vi "DAQX mod 1SDI v03.vi"(0 "resource name":refnum<k15>="PXI1Slot2", 1 "close (T)":bool=TRUE, 2 "Record Data":bool, 3 "numSamples":i32=-1, 4 "max time (s)":dbl=10.0 caption="max time", 5 "min sample rate":dbl=100000000.0, 6 "File location":path, 7 "error in":errorcluster, 8 "reference position":dbl=50.0, 9 "Additional text":string, 10 "Type of measurement":T2, 11 "Name root":string, 12 "Record TDMS":bool=TRUE caption="Enable", 13 "channel parameters":T4(array[cluster])=[{"channel name"="0", "input impedance"=0, "maximum input frequency"=30000000.0, "vertical coupling"=1, "probe attenuation"=1.0, "vertical range"=2.0, "vertical offset"=0.0, "channel enabled"=TRUE}, {"channel name"="1", "input impedance"=0, "maximum input frequency"=30000000.0, "vertical coupling"=1, "probe attenuation"=1.0, "vertical range"=2.0, "vertical offset"=0.0, "channel enabled"=TRUE}] {"input impedance" items=["1 mega ohm"=0, "50 ohms"=2]; "vertical coupling" items=["AC", "DC", "Ground"]}, 15 "reset sn":bool) -> (17 "Saving Data":bool, 18 "wfm out":waveform(dbl)[](array[waveform]), 19 "Filename Out":path, 22 "Parameters values file":string, 24 "actualSamples 0":i32, 26 "actualSamples 1":i32, 27 "error out":errorcluster caption="error out final")   [LabVIEW 2013]
doc: "Configures and acquires data from an NI-SCOPE high-speed digitizer.\n--------------------\n\nThis Express VI is configured as follows:\n\nDevice: PXI1Slot2 (PXI-5122)\nSample Rate (S/s): 100M\nRecord length: 2k\nAcquisition Mode: N Samples\nChannel 0\n - Range (V): 2\n - Offset (V): 0\n - Probe attenuation: 1\n - Coupling: \n - Input impedence: 1 \n - Bandwidth (Hz): 0\nChannel 1\n - Range (V): 2\n - Offset (V): 0\n - Probe attenuation: 1\n - Coupling: \n - Input impedence: 1 \n - Bandwidth (Hz): 0\nImmediate"
uses:
  <instrlib>/niScope/Controls/niScope vertical coupling.ctl
  Strict Type Defs/type_meas_enum.ctl
  <instrlib>/niScope/Controls/niScope timestamp type.ctl
  <instrlib>/niScope/Acquire/Fetch/niScope Multi Fetch Binary 16.vi
  <instrlib>/niScope/Acquire/Fetch/niScope Multi Fetch WDT.vi
  <instrlib>/niScope/Configure/Trigger/niScope Configure Trigger Immediate.vi
  Global VIs/shotnoise.vi
panel:
  out "Chan 1 params":T1
  out "Chan 0 params":T1
  out "file location into parameter files":path
  out "size(s)":i32
  out "actual sample rate":dbl
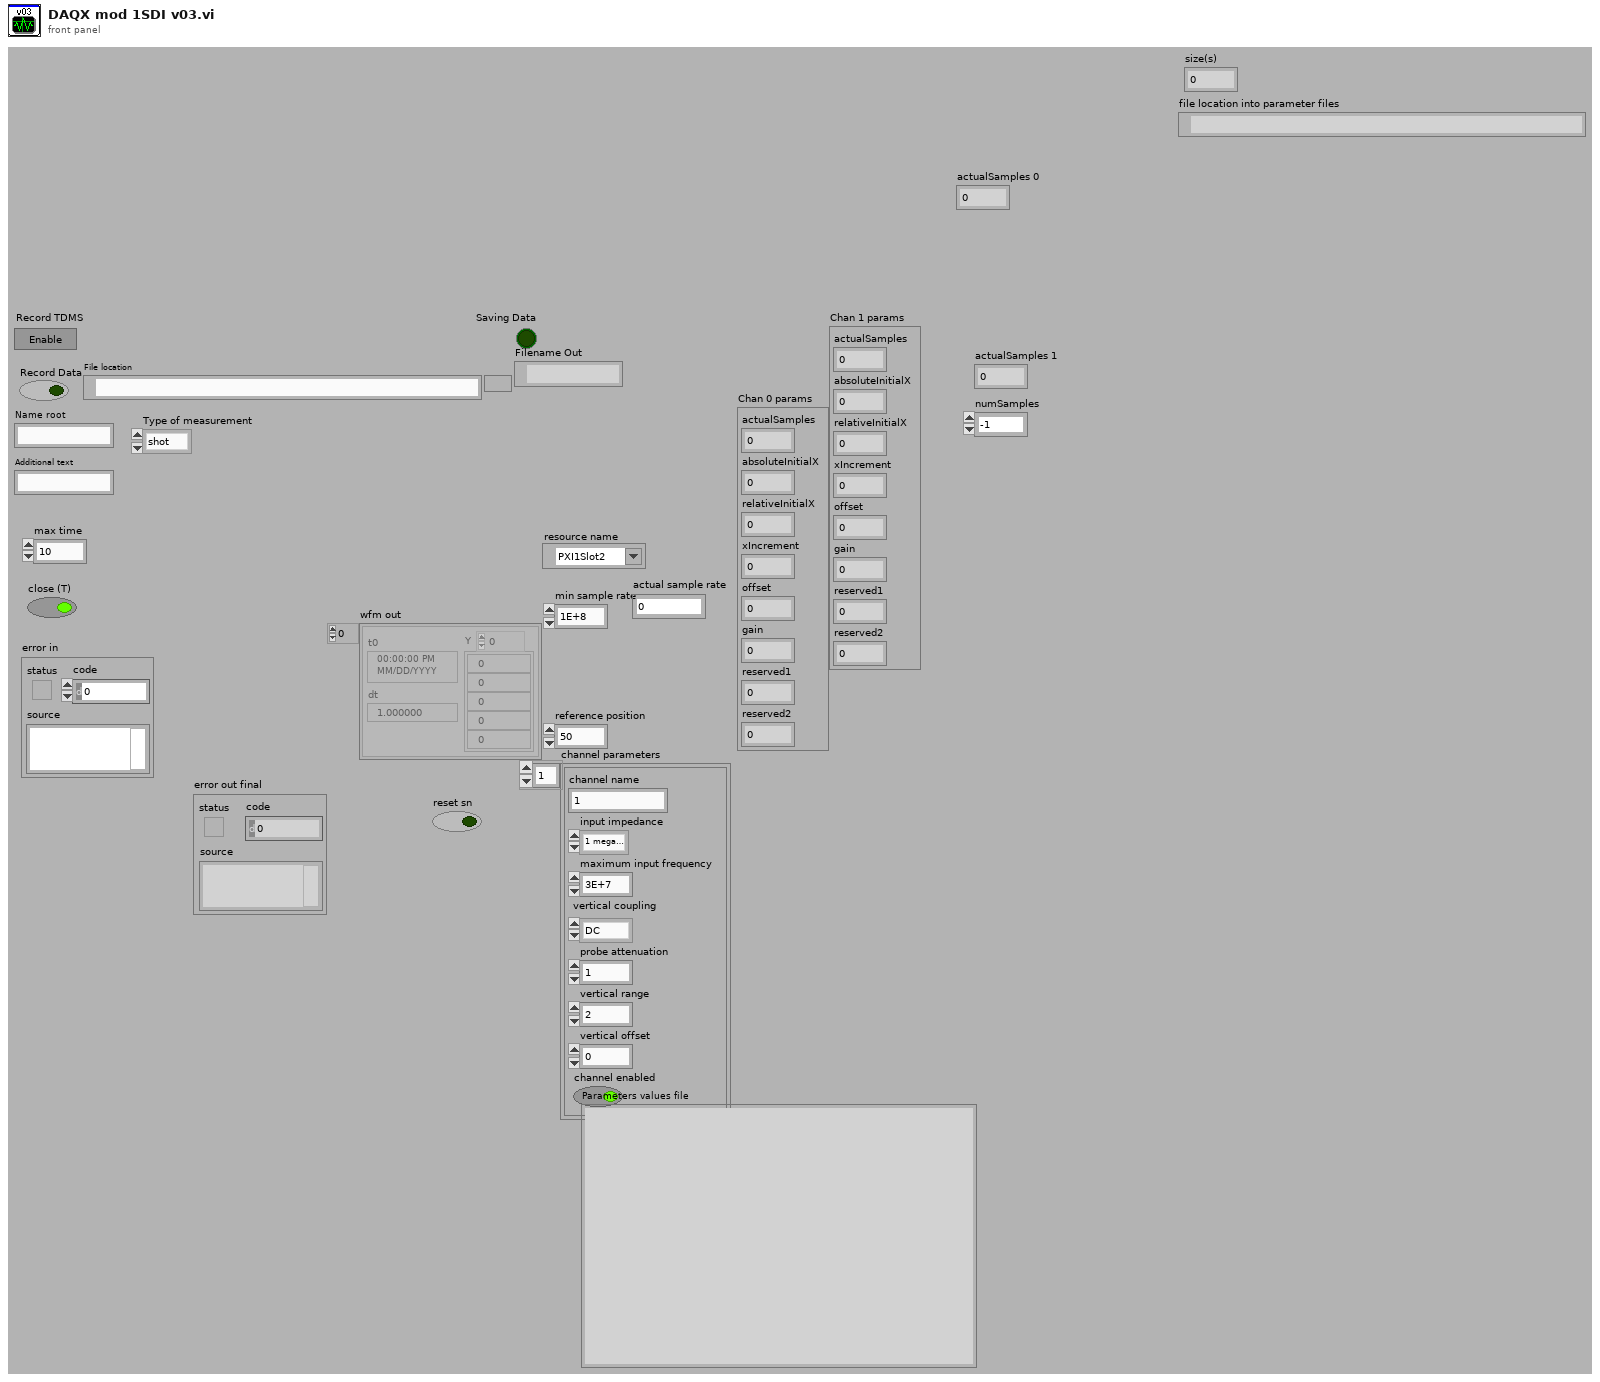
[diagram p1: front panel]
types:
  T1 = cluster{"actualSamples":i32, "absoluteInitialX":dbl, "relativeInitialX":dbl, "xIncrement":dbl, "offset":dbl, "gain":dbl, "reserved1":dbl, "reserved2":dbl}
  T2 = typedef "type_meas_enum.ctl" = enum16{"shot", "x", "p", "electronic"}
  T3 = typedef "niScope vertical coupling.ctl" = i32
  T4 = cluster{"channel name":string, "input impedance":u32, "maximum input frequency":dbl, "vertical coupling":T3, "probe attenuation":dbl, "vertical range":dbl, "vertical offset":dbl, "channel enabled":bool}[]
  T5 = typedef "niScope timestamp type.ctl" = i32
  T6 = cluster{"actualSamples":i32, "absoluteInitialX":dbl, "relativeInitialX":dbl, "xIncrement":dbl, "offset":dbl, "gain":dbl, "reserved1":dbl, "reserved2":dbl}[]
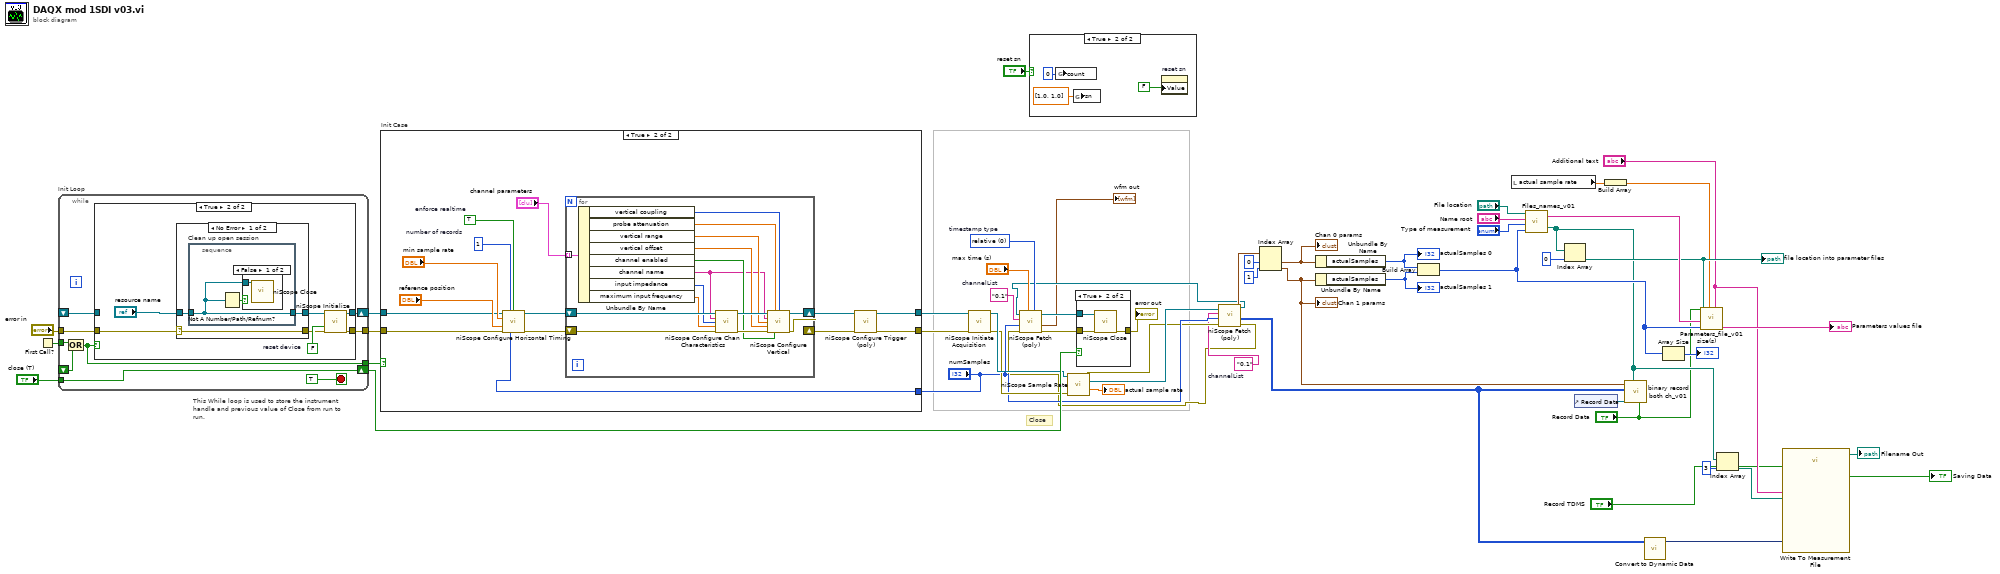
[diagram p0: block diagram]
diagram:
  w18 = "0,1"  # channelList
  w50 = T5 0 items=["relative", "absolute"]  # timestamp type
  w53 = "0,1"  # channelList
  # "This While loop is used to store the instrument handle and previous value of Close from run to run."
  # "Close"
  n1 = First Call?() -> (First Call?: T/F=w49:bool)
  n2 = while "Init Loop" {
    tunnel: w49 -> [w64]
    shift-right: [w63] -> w45
    shift-left: _ -> [w60]
    tunnel: "close (T)" -> [w63]
    shift-right: [w62] -> w48
    shift-left: _ -> [w61]
    tunnel: [w58] -> w47
    tunnel: "error in" -> [w57]
    tunnel: [w56] -> w46
    stop <- TRUE ("stopInit") stop-if-true
    n3 = Or(x=w64, y=w60) -> (x .or. y?=w56:bool)
    n4 = case "Select_Init" shown="True" w56 {
      tunnel: [w66 w71] -> w62
      tunnel: w61 -> [w66 _]
      tunnel: [w65 w70] -> w58
      tunnel: w57 -> [w65 w69]
      frame False {
      }
      frame True {
        w72 = FALSE  # reset device
        n5 = case shown="No Error" w69 {
          selector: w69 -> [w74 w80]
          tunnel: [w76 w81] -> w73
          tunnel: "resource name" -> [w75 w81]
          tunnel: [w74 w80] -> w68
          frame No Error {
            n6 = stacked-sequence "Clean up open session" {
              tunnel: w75 -> [w77]
              tunnel: [w77] -> w76
              frame #0 {
                n7 = Not A Number/Path/Refnum?(number/path/refnum=w77) -> (NaN/Path/Refnum?=w78:bool)
                n8 = case shown="False" w78 {
                  tunnel: w77 -> [w79 _]
                  frame False {
                    n9 = call <instrlib>:"niScope Close.vi"("instrument handle"=w79) -> ()  [unwired: 1 in, 14 out]
                  }
                  frame True {
                  }
                }
              }
            }
          }
          frame Error {
          }
        }
        n10 = call <instrlib>:"niScope Initialize.vi"("resource name"=w73, "reset device"=w72, "error in"=w68) -> ("instrument handle"=w71:refnum<k15>, "error out"=w70:errorcluster)  [unwired: 2 in, 9 out]
      }
    }
  }
  n11 = case "Init Case" shown="True" w46 {
    tunnel: w47 -> [w82 w88]
    tunnel: [w82 w90] -> w52
    tunnel: [w83 w91] -> w51
    tunnel: w48 -> [w83 w89]
    tunnel: "numSamples" -> [_ w84]
    frame False {
    }
    frame True {
      w96 = 1  # number of records
      w97 = TRUE  # enforce realtime
      n12 = call <instrlib>:"niScope Configure Horizontal Timing.vi"("instrument handle"=w89, "number of records"=w96, "enforce realtime"=w97, "min sample rate"="min sample rate", "reference position"="reference position", "error in"=w88, "min record length"=w84) -> ("instrument handle out"=w92:refnum<k15>, "error out"=w93:errorcluster)  [unwired: 7 out]
      n13 = for {
        shift-right: [w100] -> w85
        shift-left: w93 -> [w112]
        shift-right: [w99] -> w86
        shift-left: w92 -> [w111]
        tunnel: "channel parameters" -> [w108] mode=indexing
        n14 = Unbundle By Name(w108) -> ("vertical coupling"=w105:T3, "probe attenuation"=w104:dbl, "vertical range"=w103:dbl, "vertical offset"=w102:dbl, "channel enabled"=w101:bool, "channel name"=w98:string, "input impedance"=w106:u32, "maximum input frequency"=w107:dbl)
        n15 = call <instrlib>:"niScope Configure Chan Characteristics.vi"("instrument handle"=w111, "channels"=w98, "input impedance"=w106, "maximum input frequency"=w107, "error in"=w112) -> ("instrument handle out"=w110:refnum<k15>, "error out"=w109:errorcluster)  [unwired: 9 out]
        n16 = call <instrlib>:"niScope Configure Vertical.vi"("instrument handle"=w110, "probe attenuation"=w104, "vertical coupling"=w105, "channels"=w98, "vertical range"=w103, "vertical offset"=w102, "error in"=w109, "channel enabled"=w101) -> ("instrument handle out"=w99:refnum<k15>, "error out"=w100:errorcluster)  [unwired: 6 out]
      }
      n17 = call-poly <instrlib>:"niScope Configure Trigger (poly).vi"("instrument handle"=w86, "error in"=w85) -> ("instrument handle out"=w91:refnum<k15>, "error out"=w90:errorcluster)  [unwired: 12 out]
    }
  }
  n18 = call <instrlib>:"niScope Initiate Acquisition.vi"("instrument handle"=w51, "error in"=w52) -> ("instrument handle out"=w41:refnum<k15>, "error out"=w40:errorcluster)  [unwired: 12 out]
  n19 = case shown="True" "reset sn" {
    frame False {
    }
    frame True {
      n20 = global write "shotnoise.vi" "count"(i64 0 ("count")) -> ()
      n21 = global write "shotnoise.vi" "sn"(dbl[] [1.0, 1.0] ("sn")) -> ()
      n22 = property on="reset sn" class="Bool (strict)"("Value"=FALSE ("reset sn")) -> ()  [unwired: 2 in, 2 out]
    }
  }
  n23 = call <instrlib>:"niScope Sample Rate.vi"("instrument handle"=w41, "error in"=w40) -> ("instrument handle out"=w36:refnum<k15>, "actual sample rate"=→"actual sample rate":dbl, "error out"=w35:errorcluster)  [unwired: 11 out]
  n24 = call-poly <instrlib>:"niScope Fetch (poly).vi"("error in"=w35, "numSamples"="numSamples", "channels"=w18, "instrument handle"=w36) -> ("error out"=w16:errorcluster, "wfm"=w10:i16[][], "wfm info"=w34:T6, "instrument handle out"=w17:refnum<k15>)  [unwired: 1 in, 3 out]
  n25 = call-poly <instrlib>:"niScope Fetch (poly).vi"("timestamp Type"=w50, "timeout"="max time (s)", "error in"=w16, "numSamples"="numSamples", "channels"=w53, "instrument handle"=w17) -> ("error out"=w15:errorcluster, "wfm"=→"wfm out":waveform(dbl)[], "instrument handle out"=w39:refnum<k15>)  [unwired: 3 out]
  n26 = case shown="True" w45 {
    tunnel: w15 -> [w116 w119]
    tunnel: [w116 w118] -> w55
    tunnel: w39 -> [_ w117]
    frame False {
    }
    frame True {
      n27 = call <instrlib>:"niScope Close.vi"("instrument handle"=w117, "error in"=w119) -> ("error out"=w118:errorcluster)  [unwired: 13 out]
    }
  }
  "error out" <- w55
  n28 = Index Array(array=w34, index #1=0 ("index"), index #2=1 ("index")) -> (element #1=w31:T1, element #2=w11:T1)
  "Chan 0 params" <- w31
  "Chan 1 params" <- w11
  n29 = Unbundle By Name(w31) -> ("actualSamples"=w30:i32)
  "actualSamples 0" <- w30
  n30 = Unbundle By Name(w11) -> ("actualSamples"=w13:i32)
  "actualSamples 1" <- w13
  n31 = Build Array(w30, w13) -> (w20:i32[])
  n32 = local read "actual sample rate"() -> (w22:dbl)
  n33 = call "Files_names_v01.vi"("actualSamples\narray"=w20, "Type of\nmeasurement"="Type of measurement", "Name root"="Name root", "File location"="File location") -> ("Files path array"=w6:path[], "Files name array"=w26:string[])
  n34 = Index Array(array=w6, index=0) -> (element=w24:path)
  "file location into parameter files" <- w24
  n35 = control-ref of="Record Data"() -> (w12:refnum<vi>)
  n36 = Build Array(w22) -> (w21:dbl[])
  n37 = call "binary record both ch_v01.vi"("Record"="Record Data", "Files path array"=w6, "reference"=w12, "wfm"=w10, "Chan 1 params"=w11) -> ()  [unwired: 7 in]
  n38 = call "Convert to Dynamic Data"("2D Array"=w10) -> ("Dynamic Data Type"=w9:dynamicdata)  [unwired: 3 in]
  n39 = Array Size(array=w20) -> (size(s)=→"size(s)":i32)
  n40 = call "Parameters_file_v01.vi"("Additional text"="Additional text", "actual sample rate array"=w21, "actualSamples array"=w20, "Files name array"=w26, "File location"=w24, "Record"="Record Data") -> ("Full text"=→"Parameters values file":string)  [unwired: 3 in]
  n41 = Index Array(array=w6, index=3) -> (element=w4:path)
  n42 = call "Write To Measurement File"("Signals"=w9, "Enable"="Record TDMS", "Filename"=w4, "Comment"="Additional text") -> ("Filename Out"=→"Filename Out":path, "Saving Data"=→"Saving Data":bool)  [unwired: 13 in, 1 out]
